vi "Set Combobox Value.vi"(6 "Combo Box Ref":refnum<vi>, 7 "Data":path, 8 "error in (no error)":errorcluster, 9 "Run Mode?":bool, 10 "Indicator?":bool, 11 "Path Selector in":refnum<class "MGI Path Selector.lvclass">) -> (0 "error out":errorcluster, 3 "Path Selector out":refnum<class "MGI Path Selector.lvclass">)   [LabVIEW 2020, in "MGI Path Selector.lvclass"]
doc: "Updates the Combobox value to match the state of the XControl.\n\nAuthored by Shawn Walpole\nsupport@mooregoodideas.com\nwww.mooregoodideas.com\n\nCopyright (c) 2013, Moore Good Ideas, Inc.\n\nAll rights reserved.\n\nRedistribution and use in source and binary forms, with or without modification, are permitted provided that the following conditions are met:\n\n * Redistributions of source code must retain the above copyright notice, this list of conditions and the following disclaimer.\n * Redistributions in binary form must reproduce the above copyright notice, this list of conditions and the following disclaimer in the documentation and/or other materials provided with the distribution.\n * Neither the name of Moore Good Ideas, Inc. nor the names of its contributors may be used to endorse or promote products derived from this software without specific prior written permission.\n\nTHIS SOFTWARE IS PROVIDED BY THE COPYRIGHT HOLDERS AND CONTRIBUTORS \"AS IS\" AND ANY EXPRESS OR IMPLIED WARRANTIES, INCLUDING, BUT NOT LIMITED TO, THE IMPLIED WARRANTIES OF MERCHANTABILITY AND FITNESS FOR A PARTICULAR PURPOSE ARE DISCLAIMED. IN NO EVENT SHALL THE COPYRIGHT OWNER OR CONTRIBUTORS BE LIABLE FOR ANY DIRECT, INDIRECT, INCIDENTAL, SPECIAL, EXEMPLARY, OR CONSEQUENTIAL DAMAGES (INCLUDING, BUT NOT LIMITED TO, PROCUREMENT OF SUBSTITUTE GOODS OR SERVICES; LOSS OF USE, DATA, OR PROFITS; OR BUSINESS INTERRUPTION) HOWEVER CAUSED AND ON ANY THEORY OF LIABILITY, WHETHER IN CONTRACT, STRICT LIABILITY, OR TORT (INCLUDING NEGLIGENCE OR OTHERWISE) ARISING IN ANY WAY OUT OF THE USE OF THIS SOFTWARE, EVEN IF ADVISED OF THE POSSIBILITY OF SUCH DAMAGE."
uses:
  <userlib>/_MGI/User Interface/Path Selector XControl/Class Hierarchy/MGI Path Selector.lvclass
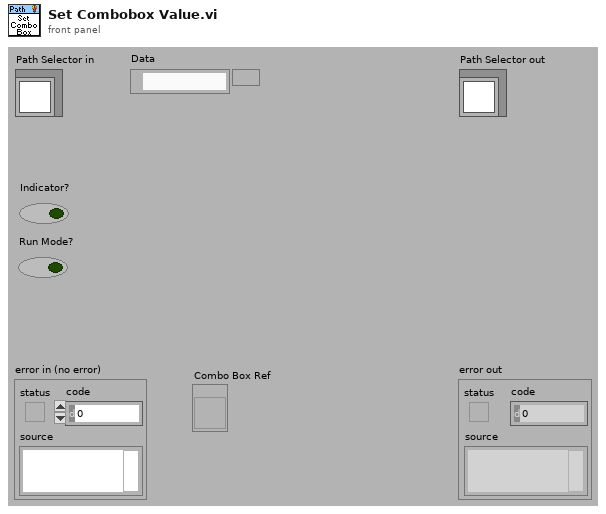
[diagram p1: front panel]
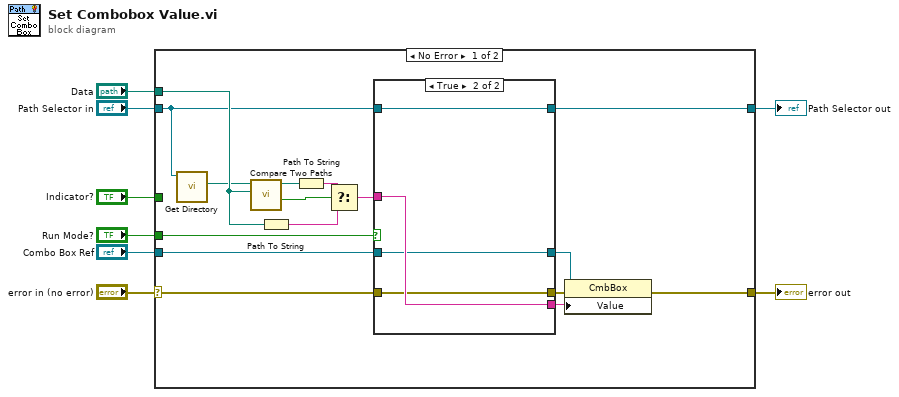
[diagram p0: block diagram]
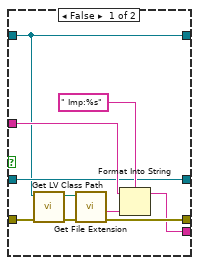
[diagram p2: hidden frame]
diagram:
  n1 = case shown="No Error" "error in (no error)" {
    selector: "error in (no error)" -> [w15 w40]
    tunnel: [w22 w40] -> w7
    tunnel: [w9 w39] -> w5
    tunnel: "Path Selector in" -> [w10 w39]
    tunnel: "Data" -> [w24 _]
    tunnel: "Combo Box Ref" -> [w12 _]
    tunnel: "Indicator?" -> [_ _]
    tunnel: "Run Mode?" -> [w16 _]
    frame No Error {
      n2 = call-dynamic "Get Directory.vi"("Path Selector in"=w10) -> ("Start Path"=w23:path)  [unwired: 9 in, 1 out]
      n3 = call <vilib>:"Compare Two Paths.vi"("Path 2"=w24, "Path 1"=w23) -> ("Path 2 Relative to Path 1?"=w21:bool, "Relative Path from 1 to 2"=w20:path)  [unwired: 6 in, 2 out]
      n4 = Path To String(path=w24) -> (string=w18:string)
      n5 = Path To String(path=w20) -> (string=w19:string)
      n6 = Select(t=w19, s=w21, f=w18) -> (s? t:f=w17:string)
      n7 = case shown="True" w16 {
        tunnel: w17 -> [w29 w38]
        tunnel: w15 -> [w31 w36]
        tunnel: [w30 w36] -> w14
        tunnel: [w28 w38] -> w13
        tunnel: w12 -> [w27 w37]
        tunnel: [w27 w37] -> w11
        tunnel: w10 -> [w26 w35]
        tunnel: [w26 w35] -> w9
        frame False {
          n8 = call <vilib>:"Get LV Class Path.vi"("error in (no error)"=w31, "object"=w26) -> ("error out"=w32:errorcluster, "class path"=w33:path)  [unwired: 8 in]
          n9 = call <vilib>:"Get File Extension.vi"("error in (no error)"=w32, "file"=w33) -> ("error out"=w30:errorcluster, "filename without extension"=w25:string)  [unwired: 5 in, 3 out]
          n10 = Format Into String(format string=" Imp:%s", initial string=w29, w25) -> (resulting string=w28:string)  [unwired: 1 in, 1 out]
        }
        frame True {
        }
      }
      n11 = property class="CmbBox"(reference=w11, error in=w14, "Value"=w13) -> (error out=w22:errorcluster)  [unwired: 1 out]
    }
    frame Error {
    }
  }
  "error out" <- w7
  "Path Selector out" <- w5
